vi "Torque.vi"() -> ()   [LabVIEW 2024]
panel:
  out "2D Picture":picture
  out "Array":cluster{dbl, dbl}[](array[cluster])
  in  "file (use dialog)":path
  out "Angle 2":dbl
  out "Angle 1":dbl
  out "T1":dbl
  out "T2":dbl
  out "T2":dynamicdata(graph) caption="Histogram"
  out "T1":dynamicdata(graph) caption="Histogram"
  out "T2":dbl(graph)
  out "T1":dbl(graph)
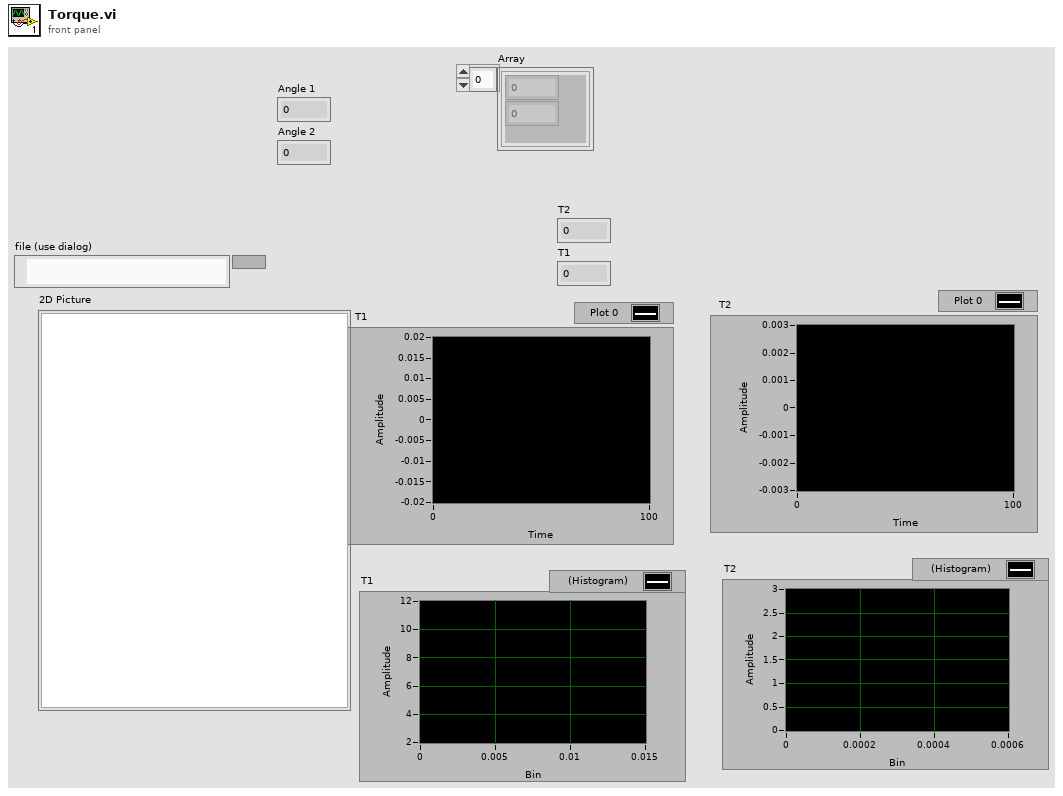
[diagram p1: front panel]
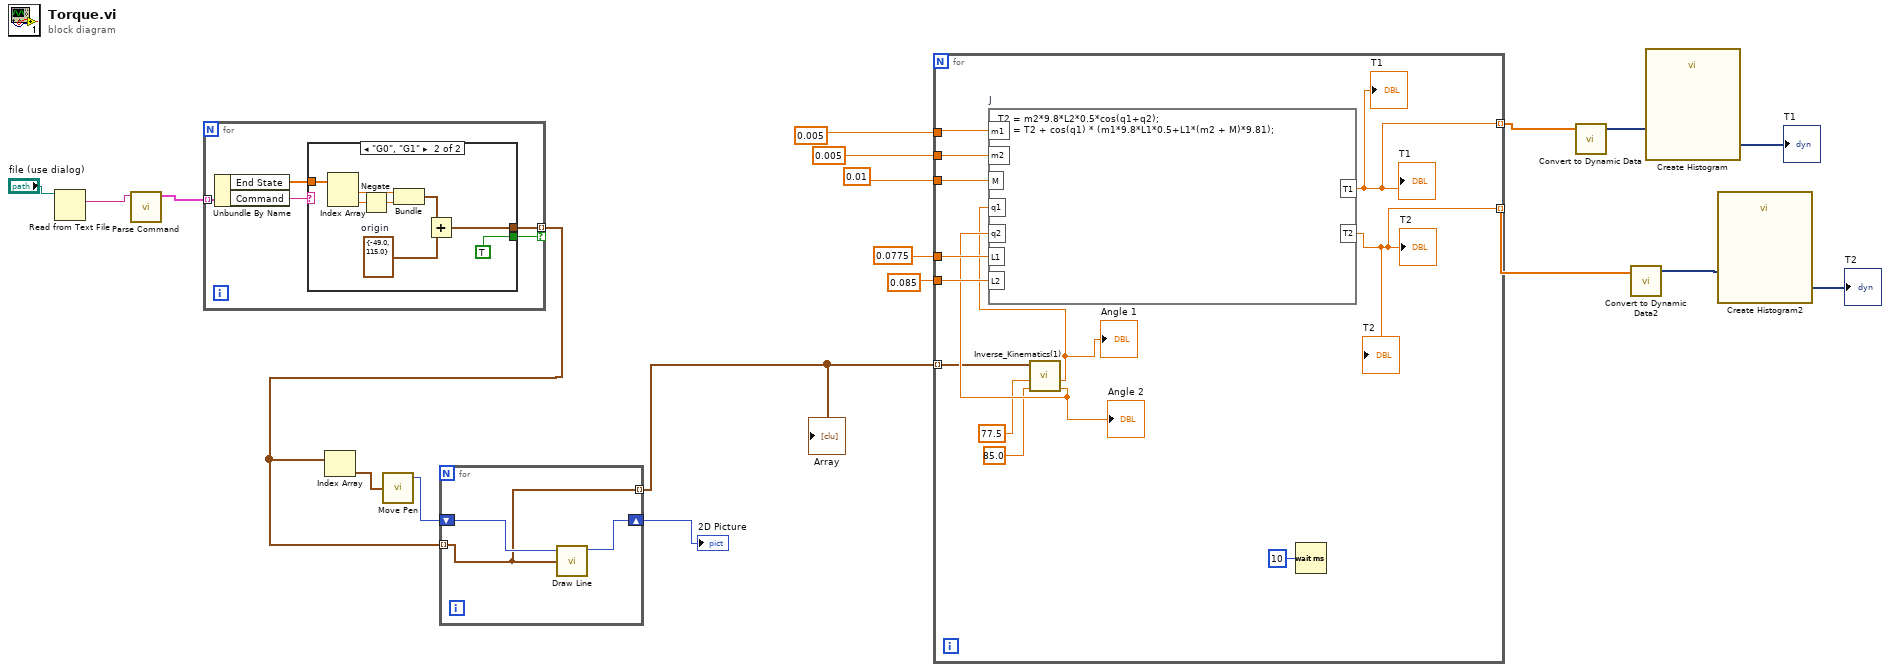
[diagram p0: block diagram]
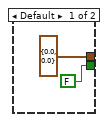
[diagram p2: hidden frame]
diagram:
  n1 = Read from Text File(file (use dialog)="file (use dialog)") -> (text=w7:string)  [unwired: 3 in, 3 out]
  n2 = call <userlib>:"Parse Command.vi"("text"=w7) -> ("cmd amd State"=w6:cluster{"Command":string, "End State":dbl[]}[])  [unwired: 8 in, 2 out]
  n3 = for {
    tunnel: w6 -> [w24] mode=indexing
    tunnel: [w21] -> w5 mode=indexing if=w20
    n4 = Unbundle By Name(w24) -> ("End State"=w22:dbl[], "Command"=w23:string)
    n5 = case shown="\"G0\", \"G1\"" w23 {
      tunnel: w22 -> [_ w34]
      tunnel: [cluster{dbl, dbl} {0.0, 0.0} w28] -> w21
      tunnel: [FALSE TRUE] -> w20
      frame Default {
      }
      frame "G0", "G1" {
        w30 = cluster{dbl, dbl} {-49.0, 115.0}  # origin
        n6 = Index Array(array=w34) -> (element #1=w32:dbl, element #2=w33:dbl)  [unwired: 2 in]
        n7 = Negate(x=w33) -> (-x=w29:dbl)
        n8 = Bundle(w32, w29) -> (w31:cluster{dbl, dbl})  [unwired: 1 in]
        n9 = Add(x=w31, y=w30) -> (x+y=w28:cluster{dbl, dbl})
      }
    }
  }
  n10 = Index Array(array=w5) -> (element=w4:cluster{dbl, dbl})  [unwired: 1 in]
  n11 = call <vilib>:"Move Pen.vi"("new position"=w4) -> ("new picture"=w3:picture)  [unwired: 4 in]
  n12 = for {
    tunnel: w5 -> [w35] mode=indexing
    shift-right: [w36] -> w1
    shift-left: w3 -> [w37]
    tunnel: [w35] -> w2 mode=indexing
    n13 = call <vilib>:"Draw Line.vi"("picture"=w37, "end point"=w35) -> ("new picture"=w36:picture)  [unwired: 7 in]
  }
  "Array" <- w2
  "2D Picture" <- w1
  n14 = for {
    tunnel: 0.005 ("Numeric") -> [w50]
    tunnel: 0.005 ("Numeric") -> [w49]
    tunnel: 0.01 ("Numeric") -> [w48]
    tunnel: 0.0775 ("Numeric") -> [w47]
    tunnel: 0.085 ("Numeric") -> [w46]
    tunnel: [w43] -> w14 mode=indexing
    tunnel: [w44] -> w12 mode=indexing
    tunnel: w2 -> [w40] mode=indexing
    n15 = call "Inverse_Kinematics(1).vi"("L 2"=85.0 ("Numeric"), "L 1"=77.5 ("Numeric"), "end effector"=w40) -> ("Angle 2"=w42:dbl, "Angle1"=w41:dbl)  [unwired: 7 in]
    "Angle 1" <- w41
    "Angle 2" <- w42
    n16 = formula code="T2 = m2*9.8*L2*0.5*cos(q1+q2);\nT1 = T2 + cos(q1) * (m1*9.8*L1*0.5+L1*(m2 + M)*9.81);" "J"("q1"=w41, "q2"=w42, "L1"=w47, "L2"=w46, "m1"=w50, "m2"=w49, "M"=w48) -> ("T1"=w43:dbl, "T2"=w44:dbl)
    "T2" <- w44
    "T1" <- w43
    "T2" <- w44
    "T1" <- w43
    n17 = Wait (ms)(milliseconds to wait=u32 10) -> ()  [unwired: 1 out]
  }
  n18 = call "Convert to Dynamic Data"("Array"=w14) -> ("Dynamic Data Type"=w13:dynamicdata)  [unwired: 3 in]
  n19 = call "Convert to Dynamic Data2"("Array"=w12) -> ("Dynamic Data Type"=w11:dynamicdata)  [unwired: 3 in]
  n20 = call "Create Histogram"("Signal"=w13) -> ("Histogram"=→"T1":dynamicdata)  [unwired: 9 in, 1 out]
  n21 = call "Create Histogram2"("Signal"=w11) -> ("Histogram"=→"T2":dynamicdata)  [unwired: 9 in, 1 out]
